vi "arange (SubVI).vi"(9 "# Steps":i32, 10 "stop":ext, 11 "start":ext) -> (3 "Array":ext[](array[numeric]))   [LabVIEW 2022 SP3]
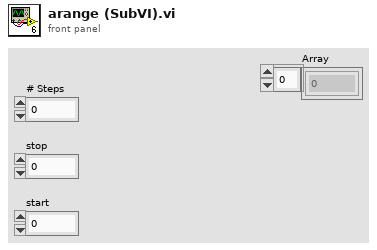
[diagram p1: front panel]
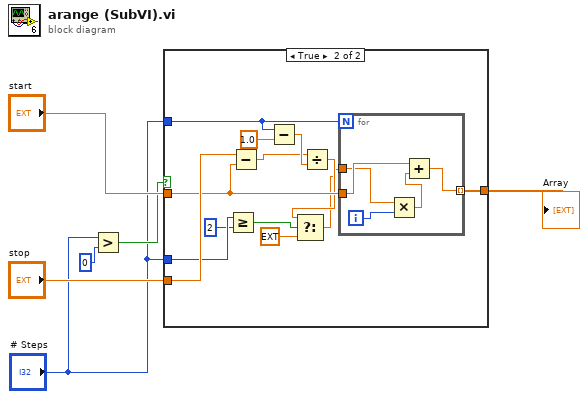
[diagram p0: block diagram]
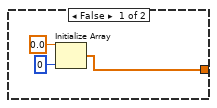
[diagram p2: hidden frame]
diagram:
  n1 = Greater?(x="# Steps", y=0) -> (0:w2:bool)
  n2 = case shown="True" w2 {
    tunnel: "# Steps" -> [_ w20]
    tunnel: "start" -> [_ w16]
    tunnel: "stop" -> [_ w17]
    tunnel: [w9 w18] -> w4
    tunnel: "# Steps" -> [_ w12]
    frame False {
      n3 = Initialize Array(0.0 ("element"), 0 ("dimension size")) -> (w9:dbl[])
    }
    frame True {
      n4 = Greater Or Equal?(x=w12, y=2) -> (x >= y?=w11:bool)
      n5 = Subtract(x=w17, y=w16) -> (x-y=w19:ext)
      n6 = Subtract(x=w20, y=1.0) -> (x-y=w22:dbl)
      n7 = Divide(x=w19, y=w22) -> (x/y=w15:ext)
      n8 = Select(t=w15, s=w11, f=ext 1.0) -> (s? t:f=w14:ext)
      n9 = for {
        N: w20 -> [_]
        tunnel: w16 -> [w27]
        tunnel: [w26] -> w18 mode=indexing
        tunnel: w14 -> [w23]
        i -> [w25]
        n10 = Multiply(x=w23, y=w25) -> (x*y=w24:ext)
        n11 = Add(x=w27, y=w24) -> (x+y=w26:ext)
      }
    }
  }
  "Array" <- w4
